vi "Get PC Info.vi"(8 "error in (no error)":errorcluster) -> (0 "error out":errorcluster, 2 "PC ID":string, 3 "PC Name":string)   [LabVIEW 2020]
uses:
  <vilib>/Utility/sysdir.llb/System Directory Type.ctl
  <vilib>/regexp/Match Regular Expression.xnode
  kernel32.dll
panel:
  out "resulting string":string
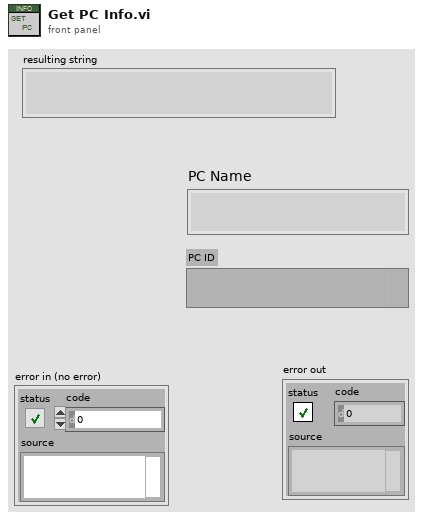
[diagram p1: front panel]
types:
  T1 = typedef "System Directory Type.ctl" = i32
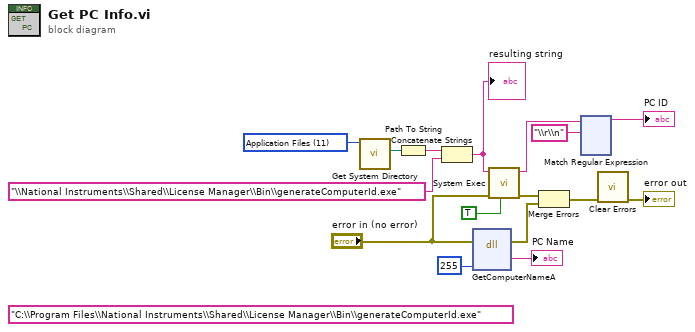
[diagram p0: block diagram]
diagram:
  w5 = T1 11 items=["User Home"=0, "User Desktop"=1, "User Documents"=2, "User Application Data"=3, "User Preferences"=4, "User Temporary"=5, "Public Documents"=6, "Public Application Data"=7, "Public Preferences"=8, "Public Cache"=13, "System Core Libraries"=9, "System Installed Libraries"=10, "Application Files"=11, "Boot Volume Root"=12] ("system directory type")
  (unwired) "C:\\Program Files\\National Instruments\\Shared\\License Manager\\Bin\\generateComputerId.exe"
  n1 = call <vilib>:"Get System Directory.vi"("system directory type"=w5) -> ("system directory"=w3:path)  [unwired: 10 in]
  n2 = Path To String(path=w3) -> (string=w4:string)
  n3 = Concatenate Strings(w4, "\\National Instruments\\Shared\\License Manager\\Bin\\generateComputerId.exe") -> (w2:string)
  "resulting string" <- w2
  n4 = dll-call lib="kernel32.dll" fn="GetComputerNameA"(error in="error in (no error)", "lpnSize"=u32 255) -> (error out=w12:errorcluster, "lpbuffer"=→"PC Name":string)  [unwired: 5 in, 1 out]
  n5 = call <vilib>:"System Exec.vi"("run minimized? (F)"=TRUE, "error in (no error)"="error in (no error)", "command line"=w2) -> ("error out"=w13:errorcluster, "standard output"=w8:string)  [unwired: 5 in, 2 out]
  n6 = Merge Errors(w13, w12) -> (w11:errorcluster)
  n7 = xnode "Match Regular Expression"("input string"=w8, "regular expression"="\\r\\n" ("regular expression (\"\")")) -> ("before match"=→"PC ID":string)  [unwired: 4 in, 4 out]
  n8 = call <vilib>:"Clear Errors.vi"("error in (no error)"=w11) -> ("error out"=→"error out":errorcluster)  [unwired: 5 in, 1 out]
